vi "北斗显示界面.vi"() -> ()   [LabVIEW 2016, in "环境动力监测库.lvlib" / "NMEA.lvlib"]
uses:
  NMEA.lvlib
  NMEA_GPVTG-data.ctl
  NMEA_Mode.ctl
  NMEA_GPRMC-data.ctl
  NMEA_LatitudeDirection.ctl
  NMEA_LongitudeDirection.ctl
  NMEA_GPGGA-data.ctl
  NMEA_GPS-Quality.ctl
  <vilib>/Utility/miscctls.llb/LVPointTypeDef.ctl
  <vilib>/Instr/_visa.llb/VISA Configure Serial Port (Instr).vi
  <vilib>/Utility/config.llb/NI_LVConfig.lvlib
  <vilib>/ptbypt/NI_PtbyPt.lvlib
panel:
  out "波特率":u32
  out "串口":string
  in  "收方地址设定值":string
  in  "发送测试":bool
  in  "移位报警设定值":dbl=1000.0
  out "浮标定位点":cluster{"纬度":dbl, "经度":dbl}
  out "定位状态":bool
  in  "配置":bool
  out "Coordinates":picture
  in  "reset odometer":bool
  out "方位角 (deg)":dbl(knob) scale=0.0..360.0
  out "偏移量/米":dbl format="%#.2f"
  out "水平运动速度 (km/h)":dbl(knob) scale=0.0..180.0
  out "海拔":dbl format="%.2f"
  out "纬度":dbl
  out "经度":dbl
  out "时间":timestamp format="%<%H:%M:%S>T"
  out "日期":timestamp format="%<%Y/%m/%d>T"
  out "$GPGGA-message_OUT":T1={"TimeStamp"=timestamp(0 s since 1904-01-01), "Latitude"=0.0, "Latitude-Direction"=enum."", "Longitude"=1.0, "Longitude-Direction"=enum."", "GPS-Quality"=enum."GPS fix (SPS)", "Number of Satellites"=0, "Horizontal Dilution of Precision"=0.0, "Altitude above Mean-Sea-Level"=0.0, "Geoidal separation"=0.0, "Time since last DGPS update"=0.0, "DGPS reference station ID"=0} {"Time since last DGPS update" format="%.02f [s]"; "Geoidal separation" format="%.02f [m]"; "Altitude above Mean-Sea-Level" format="%.02f [m]"; "Horizontal Dilution of Precision" format="%.02f [HDOP]"; "Longitude" format="%0.4f [long]"; "Latitude" format="%.04f [lat]"; "TimeStamp" format="%<%.2X>T"}
  out "$GPRMC-message_OUT":T5={"TimeStamp"=timestamp(0 s since 1904-01-01), "Validity"=FALSE, "Latitude"=0.0, "Latitude-Direction"=enum."North", "Longitude"=0.0, "Longitude-Direction"=enum."East", "Speed in knots"=0.0, "True course"=0.0, "Date Stamp"=timestamp(0 s since 1904-01-01), "Magnetic Variation (East/West)"=0.0} {"Magnetic Variation (East/West)" format="%.02f [deg]"; "Date Stamp" format="%<%x>T"; "True course" format="%.02f [deg]"; "Speed in knots" format="%.02f [kts]"; "Longitude" format="%0.4f [long]"; "Latitude" format="%.04f [lat]"; "TimeStamp" format="%<%.2X>T"}
  out "$GPVTG-message_OUT":T6={"True Course over Ground"=0.0, "Magnetic Course over Ground"=0.0, "Speed over Ground in knots"=0.0, "Speed over Ground in km/h"=1.0, "Mode"=""} {"Speed over Ground in km/h" format="%.02f [km/h]"; "Speed over Ground in knots" format="%.02f [kts]"; "Magnetic Course over Ground" format="%.02f [deg]"; "True Course over Ground" format="%.02f [deg]"}
  out "Raw data GPS":string
  in  "Stop":bool
  # "米"
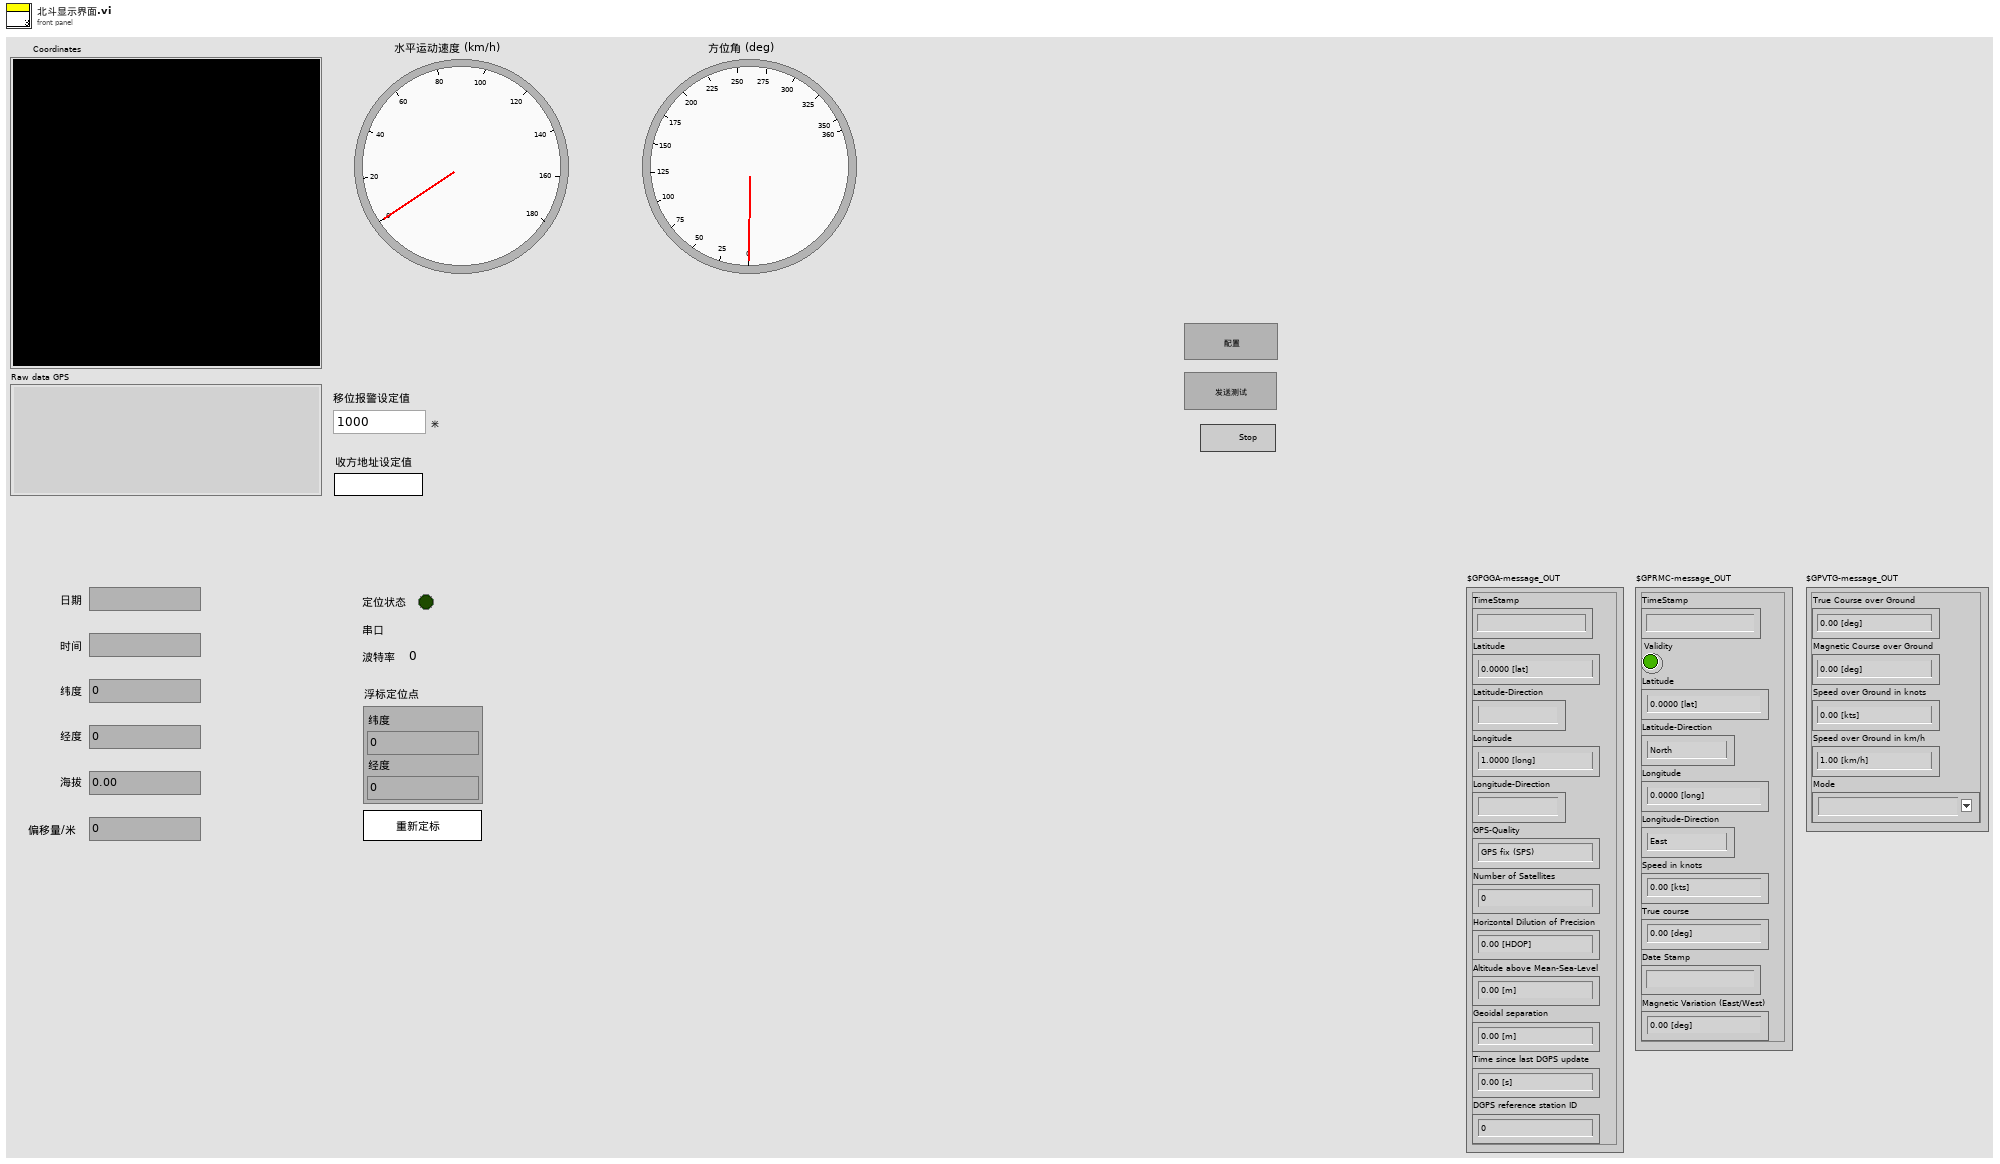
[diagram p1: front panel]
types:
  T1 = typedef "环境动力监测库.lvlib/NMEA.lvlib/NMEA_GPGGA-data.ctl" = cluster{"TimeStamp":timestamp, "Latitude":dbl, "Latitude-Direction":T2, "Longitude":dbl, "Longitude-Direction":T3, "GPS-Quality":T4, "Number of Satellites":i32, "Horizontal Dilution of Precision":dbl, "Altitude above Mean-Sea-Level":dbl, "Geoidal separation":dbl, "Time since last DGPS update":dbl, "DGPS reference station ID":i32}
  T2 = typedef "环境动力监测库.lvlib/NMEA.lvlib/NMEA_LatitudeDirection.ctl" = enum16{"", "North", "South"}
  T3 = typedef "环境动力监测库.lvlib/NMEA.lvlib/NMEA_LongitudeDirection.ctl" = enum16{"", "East", "West"}
  T4 = typedef "环境动力监测库.lvlib/NMEA.lvlib/NMEA_GPS-Quality.ctl" = enum16{"Invalid", "GPS fix (SPS)", "DGPS fix", "PPS fix", "Real Time Kinematic", "Float RTK", "estimated", "Manual input mode", "Simulation mode"}
  T5 = typedef "环境动力监测库.lvlib/NMEA.lvlib/NMEA_GPRMC-data.ctl" = cluster{"TimeStamp":timestamp, "Validity":bool, "Latitude":dbl, "Latitude-Direction":T2, "Longitude":dbl, "Longitude-Direction":T3, "Speed in knots":dbl, "True course":dbl, "Date Stamp":timestamp, "Magnetic Variation (East/West)":dbl}
  T6 = typedef "环境动力监测库.lvlib/NMEA.lvlib/NMEA_GPVTG-data.ctl" = cluster{"True Course over Ground":dbl, "Magnetic Course over Ground":dbl, "Speed over Ground in knots":dbl, "Speed over Ground in km/h":dbl, "Mode":T7}
  T7 = typedef "环境动力监测库.lvlib/NMEA.lvlib/NMEA_Mode.ctl" = string
  T8 = cluster{"监测项描述:输出":string, "连接方式":enum16{"串口", "TCP"}, "端口":string, "IP address:":string, "Port:":string, "站号":u64, "传感器型号":string, "波特率":u64, "data bits":u64, "停止位":u16, "奇偶校验":u16}
  T9 = typedef "LVPointTypeDef.ctl" = cluster{"Horizontal":i16, "Vertical":i16}
  T10 = typedef "NI_LVConfig.lvlib/Config Data RefNum.ctl" = refnum<k1>
  T11 = enum32{"invalid app kind", "Development System", "Run Time System", "Student Edition", "Embedded LabVIEW", "Evaluation", "Custom"}
  T12 = cluster{"电压":dbl, "温度":dbl, "湿度":dbl, "GPS":cluster{"经度":dbl, "纬度":dbl}, "BD":cluster{"经度":dbl, "纬度":dbl}}
  T13 = typedef "LVDateTimeRec.ctl" = cluster{"秒数的小数部分":dbl, "秒":i32, "分":i32, "时":i32, "日":i32, "月":i32, "年":i32, "天数（周）":i32, "天数（年）":i32, "DST":i32}
  T14 = cluster{"温湿度":cluster{"状态":bool, "温度:":sgl, "湿度:":sgl, "详情  ":bool}, "空调":cluster{"状态":bool, "机柜温度:":sgl, "压缩机:":enum16{"停止", "运行"}, "电加热:":enum16{"停止", "运行"}, "详情  ":bool}, "排气扇":cluster{"排气扇:":enum16{"关闭", "打开"}, "详情  ":bool}, "冰箱":cluster{"冰箱:":enum16{"关闭", "打开"}, "详情  ":bool}}
  T15 = cluster{"市电":cluster{"状态":bool, "电压:":u16, "电流：":dbl, "详情  ":bool}, "UPS":cluster{"状态":bool, "输入电压:":sgl, "输出电压:":sgl, "电池电量:":u8, "电量":u16, "详情  ":bool}, "蓄电池12V":cluster{"状态":bool, "电压:":sgl, "电流:":sgl, "电池电量:":u8, "电量":u16, "详情  ":bool}, "蓄电池24V":cluster{"状态":bool, "电压:":sgl, "电流:":sgl, "电池电量:":u8, "电量":u16, "详情  ":bool}}
  T16 = cluster{"网络状态":bool, "电源管理":cluster{"电源管理":bool, "氨氮电源":bool, "总磷电源":bool, "总氮电源":bool, "多参数电源":bool, "CODMn电源":bool, "CODCr电源":bool, "灯带电源":bool, "照明电源":bool}, "北斗-GPS":cluster{"北斗":cluster{"经度:":sgl, "纬度:":sgl, "北斗监测":bool}, "GPS":cluster{"经度:":sgl, "纬度: ":sgl, "GPS监测":bool}}}
  T17 = cluster{"漏水监测输出":cluster{"漏水监测告警":bool, "告警内容":string}, "门禁监测输出":cluster{"门禁监测告警":bool, "告警内容":string}, "门禁监测输出2":cluster{"门禁监测告警":bool, "告警内容":string}, "温湿度监测输出":cluster{"温湿度监测告警":bool, "告警内容":string}, "烟雾监测输出":cluster{"烟雾监测告警":bool, "告警内容":string}, "空调监测输出":cluster{"空调监测告警":bool, "告警内容":string}, "自动重合闸输出":cluster{"自动重合闸告警":bool, "告警内容":string}, "红外入侵输出":cluster{"红外入侵告警":bool, "告警内容":string}, "振动输出":cluster{"振动告警":bool, "告警内容":string}, "UPS输出":cluster{"UPS告警":bool, "告警内容":string}, "蓄电池输出":cluster{"蓄电池告警":bool, "告警内容":string}, "蓄电池输出2":cluster{"蓄电池告警":bool, "告警内容":string}, "GPS输出":cluster{"定位告警":bool, "告警内容":string}, "北斗输出":cluster{"定位告警":bool, "告警内容":string}, "气象输出":cluster{"气象告警":bool, "告警内容":string}}
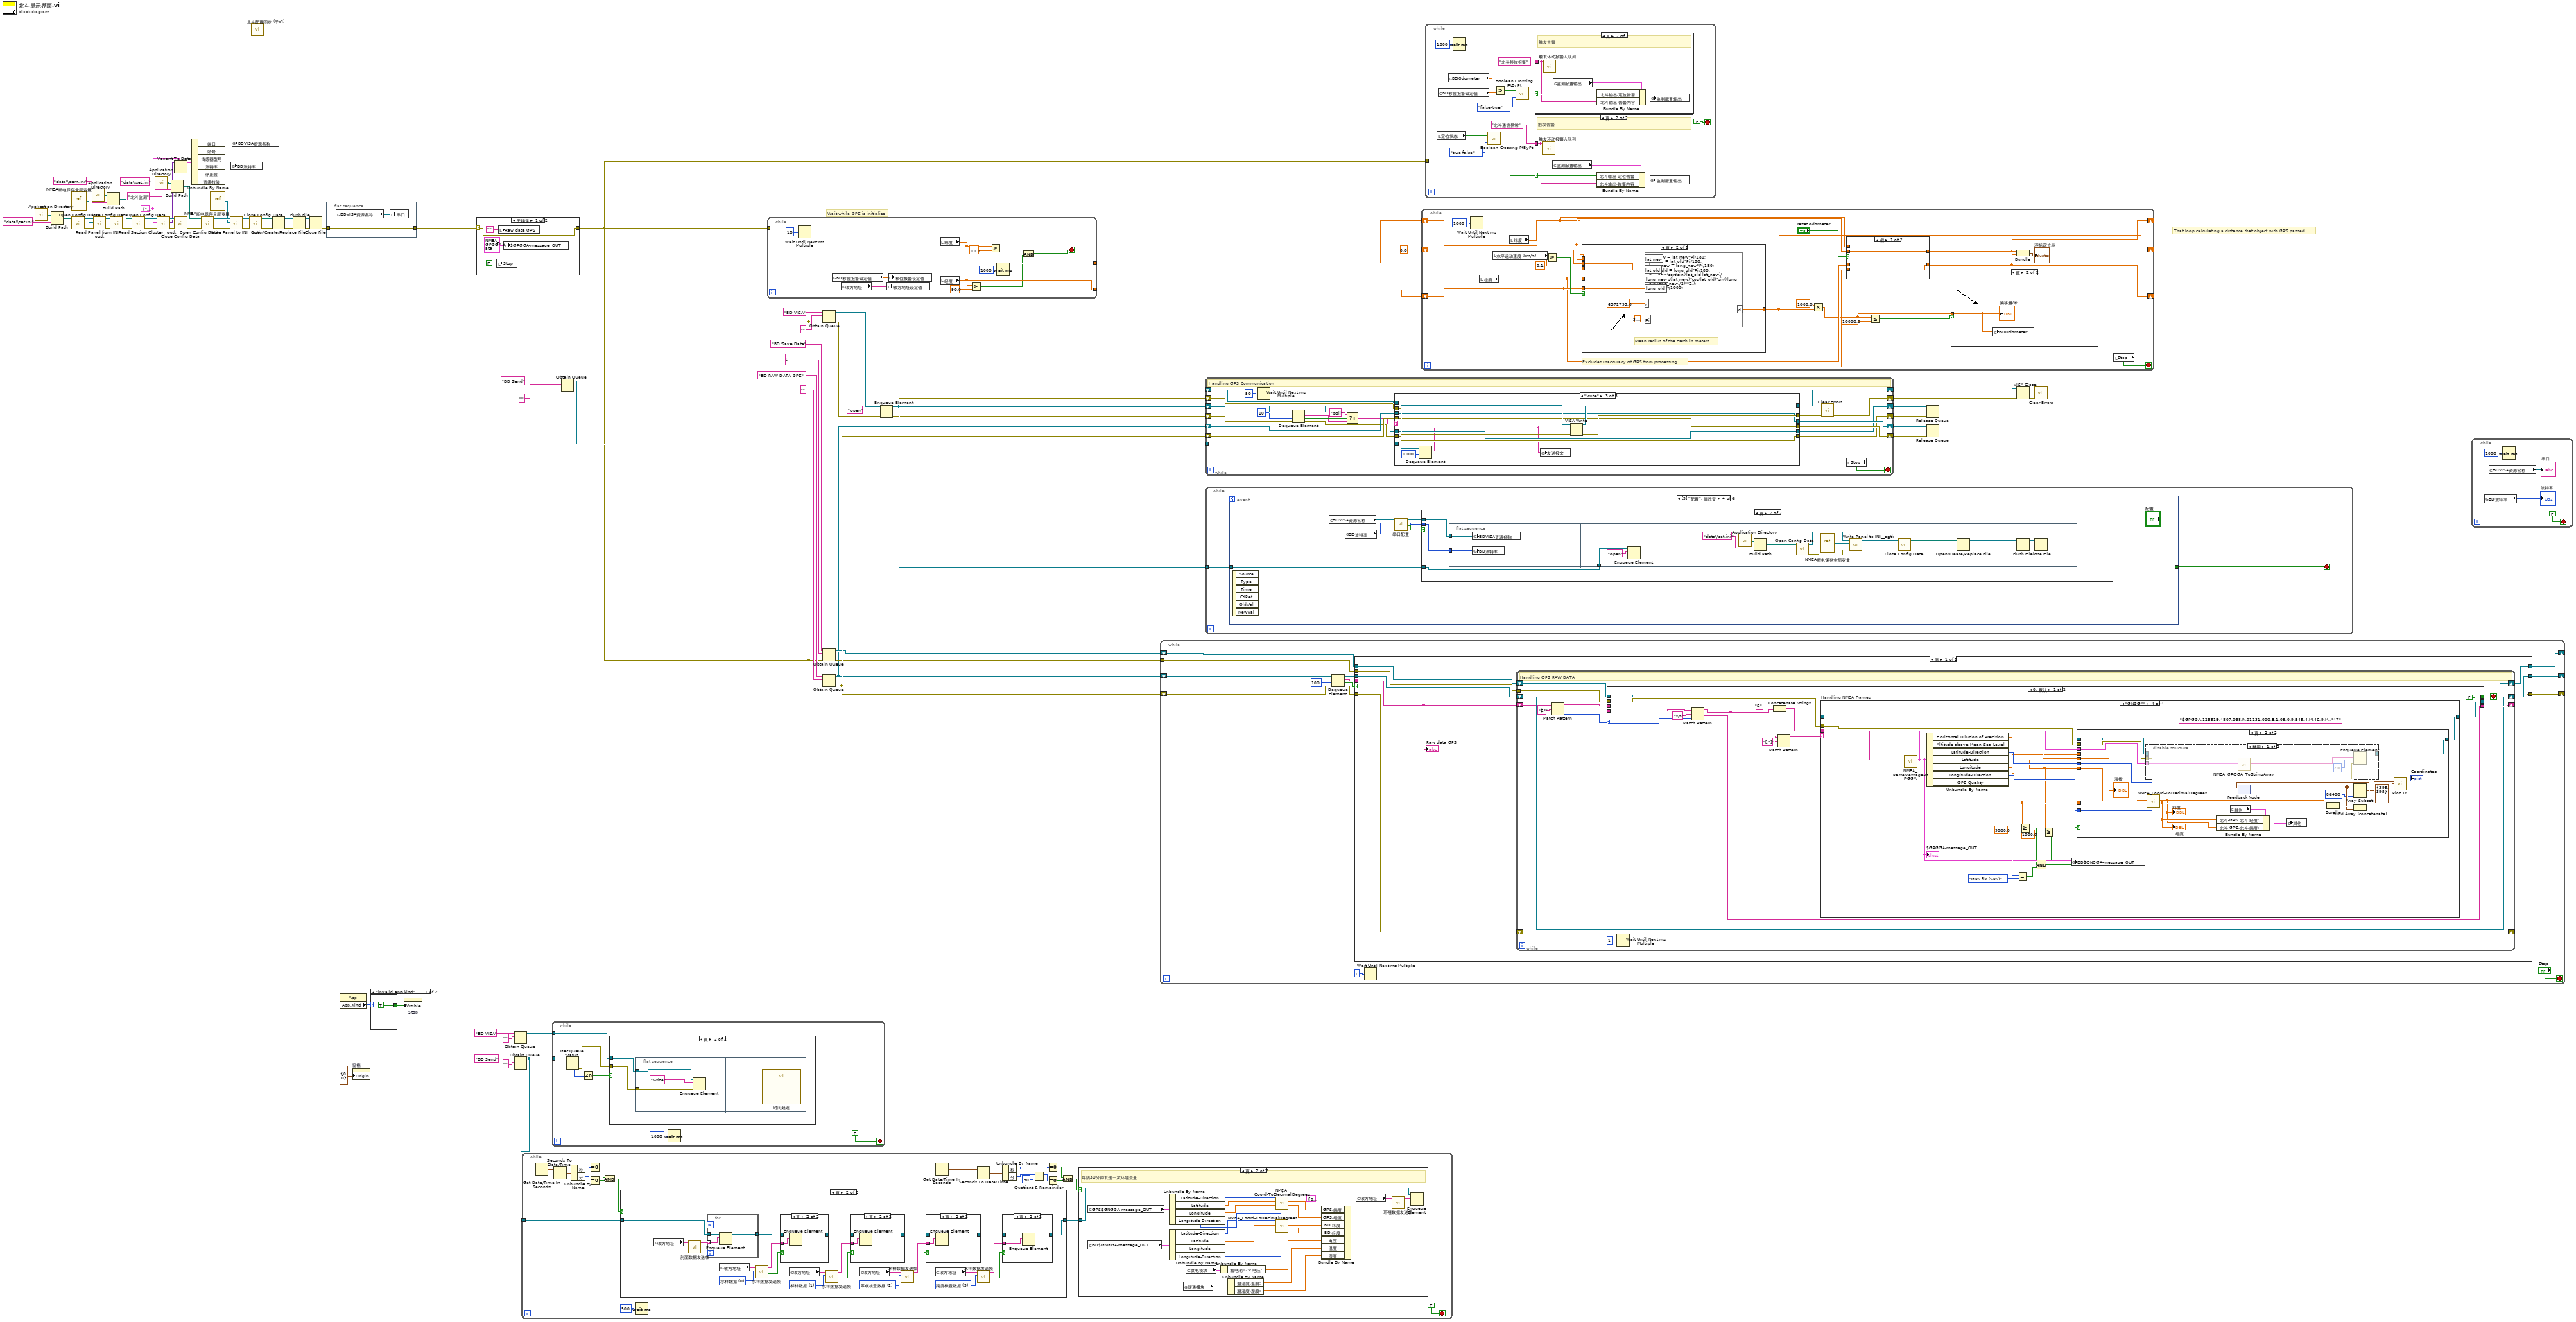
[diagram p0: block diagram]
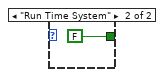
[diagram p11: hidden frame]
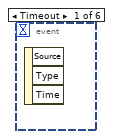
[diagram p12: hidden frame]
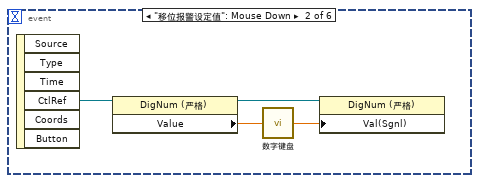
[diagram p13: hidden frame]
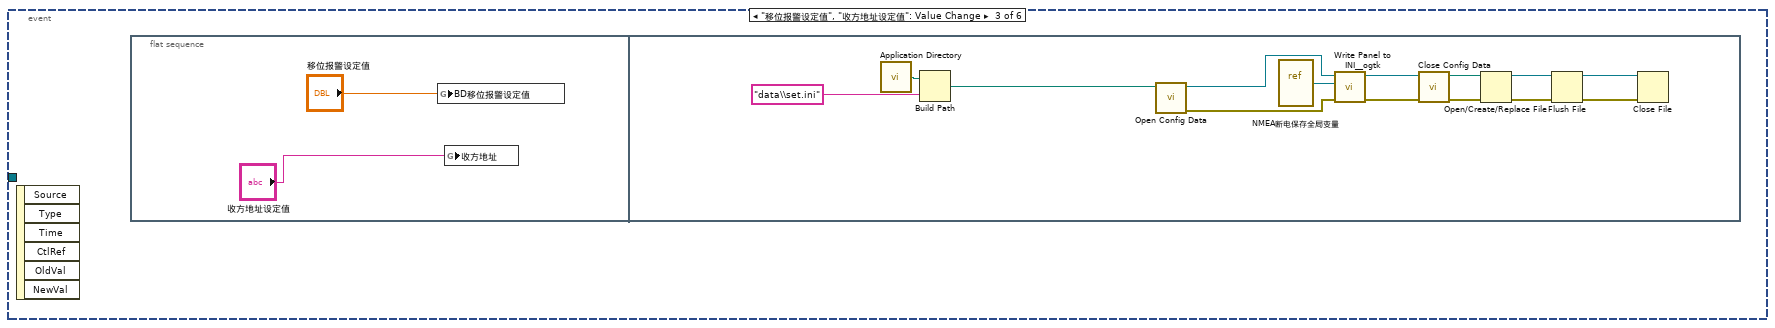
[diagram p14: hidden frame]
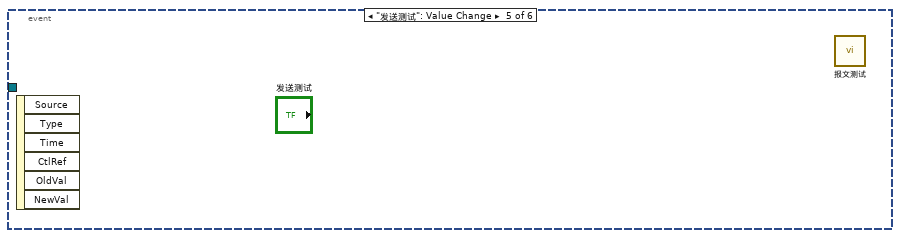
[diagram p16: hidden frame]
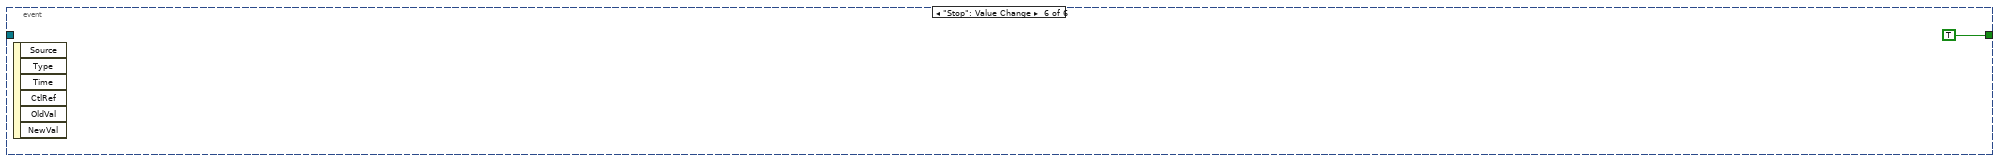
[diagram p17: hidden frame]
diagram:
  w22 = T8 {"监测项描述:输出"="", "连接方式"=enum."串口", "端口"="", "IP address:"="", "Port:"="", "站号"=19200, "传感器型号"="", "波特率"=19200, "data bits"=8, "停止位"=10, "奇偶校验"=0} ("输入簇")
  # "That loop calculating a distance that object with GPS passed"
  # "Wait while GPS is initialize"
  n1 = call <vilib>:"Application Directory.vi"() -> ("Application Directory"=w35:path)
  n2 = Build Path(base path=w35, name or relative path="data\\set.ini" ("名称或相对路径")) -> (appended path=w34:path)
  n3 = vi-ref "NMEA断电保存全局变量.vi"() -> (w33:refnum<vi>)
  n4 = call <vilib>:"Open Config Data.vi"("configuration file path"=w34) -> ("error out"=w38:errorcluster, "refnum"=w37:T10)  [unwired: 8 in, 1 out]
  n5 = call <vilib>:"Application Directory.vi"() -> ("Application Directory"=w29:path)
  n6 = call <userlib>:"Read Panel from INI__ogtk.vi"("error in (no error)"=w38, "VI ref"=w33, "refnum"=w37) -> ("error out"=w40:errorcluster, "refnum out"=w39:T10)  [unwired: 7 in]
  n7 = Build Path(base path=w29, name or relative path="data\\pem.ini" ("名称或相对路径")) -> (appended path=w30:path)
  n8 = call <vilib>:"Close Config Data.vi"("error in (no error)"=w40, "refnum"=w39) -> ("error out"=w4:errorcluster)  [unwired: 8 in, 1 out]
  n9 = call <vilib>:"Open Config Data.vi"("error in (no error)"=w4, "configuration file path"=w30) -> ("error out"=w31:errorcluster, "refnum"=w32:T10)  [unwired: 7 in, 1 out]
  n10 = call <vilib>:"Application Directory.vi"() -> ("Application Directory"=w18:path)
  n11 = call <userlib>:"Read Section Cluster__ogtk.vi"("section (optional)"="北斗监测", "error in (no error)"=w31, "Section Formatted Cluster Type"=w22, "refnum"=w32) -> ("error out"=w25:errorcluster, "Section Formatted Cluster"=w24:variant, "dup refnum"=w26:T10)  [unwired: 3 in, 2 out]
  n12 = Build Path(base path=w18, name or relative path="data\\set.ini" ("名称或相对路径")) -> (appended path=w19:path)
  n13 = Variant To Data(type=w22, Variant=w24) -> (data=w23:T8)  [unwired: 1 in, 1 out]
  n14 = call <vilib>:"Close Config Data.vi"("error in (no error)"=w25, "refnum"=w26) -> ("error out"=w3:errorcluster)  [unwired: 8 in, 1 out]
  n15 = Unbundle By Name(w23) -> ("端口"=w21:string, "波特率"=w20:u64)  [unwired: 4 out]
  n16 = call <vilib>:"Open Config Data.vi"("error in (no error)"=w3, "configuration file path"=w19) -> ("error out"=w15:errorcluster, "refnum"=w16:T10)  [unwired: 7 in, 1 out]
  n17 = vi-ref "NMEA断电保存全局变量.vi"() -> (w12:refnum<vi>)
  n18 = call <userlib>:"Write Panel to INI__ogtk.vi"("error in (no error)"=w15, "VI ref"=w12, "refnum"=w16) -> ("error out"=w13:errorcluster, "refnum out"=w14:T10)  [unwired: 7 in]
  n19 = global write "NMEA断电保存全局变量.vi" "BD波特率"(w20) -> ()
  n20 = global write "NMEA断电保存全局变量.vi" "BDVISA资源名称"(w21) -> ()
  n21 = call <vilib>:"Close Config Data.vi"("error in (no error)"=w13, "refnum"=w14) -> ("error out"=w11:errorcluster, "file path"=w10:path)  [unwired: 8 in]
  n22 = call "北斗配置同步 (子VI).vi"() -> ()  [unwired: 12 in]
  n23 = Open/Create/Replace File(file path (use dialog)=w10, error in=w11) -> (refnum out=w8:refnum<file>, error out=w9:errorcluster)  [unwired: 4 in, 1 out]
  n24 = Flush File(refnum=w8, error in=w9) -> (refnum out=w6:refnum<file>, error out=w7:errorcluster)
  n25 = Close File(refnum=w6, error in=w7) -> (error out=w5:errorcluster)  [unwired: 1 out]
  n26 = flat-sequence {
    tunnel: w5 -> [w78]
    tunnel: [w78] -> w2
    frame #0 {
      n27 = global read "NMEA断电保存全局变量.vi" "BDVISA资源名称"() -> (w79:refnum<visa-resource-name>)
      n28 = local write "串口"(w79) -> ()
    }
  }
  n29 = property class="App"() -> ("App.Kind"=w60:T11)  [unwired: 2 in, 2 out]
  n30 = property on="窗格" class="Pane"("Origin"=T9 {"Horizontal"=0, "Vertical"=0} ("原点")) -> ()  [unwired: 2 in, 2 out]
  n31 = case shown="\"invalid app kind\", 默认" w60 {
    tunnel: [TRUE ("可见") FALSE ("可见")] -> w59
    frame "invalid app kind", Default {
    }
    frame "Run Time System" {
    }
  }
  n32 = property on="Stop" class="Bool (严格)"("Visible"=w59) -> ()  [unwired: 2 in, 2 out]
  n33 = case shown="无错误" w2 {
    selector: w2 -> [w84 w86]
    tunnel: [w84 w86] -> w1
    frame No Error {
      n34 = local write "Stop"(FALSE ("STOP")) -> ()
      n35 = local write "Raw data GPS"("") -> ()
      n36 = local write "$GPGGA-message_OUT"(T1 {"TimeStamp"=timestamp(0 s since 1904-01-01), "Latitude"=0.0, "Latitude-Direction"=enum."North", "Longitude"=0.0, "Longitude-Direction"=enum."East", "GPS-Quality"=enum."Invalid", "Number of Satellites"=0, "Horizontal Dilution of Precision"=0.0, "Altitude above Mean-Sea-Level"=0.0, "Geoidal separation"=0.0, "Time since last DGPS update"=0.0, "DGPS reference station ID"=0} ("GPGGA-data")) -> ()
    }
    frame Error {
    }
  }
  n37 = Obtain Queue(name (unnamed)="BD VISA" ("名称（未命名）"), element data type="" ("名称（未命名）")) -> (queue out=w41:refnum<queue>)  [unwired: 3 in, 2 out]
  n38 = Obtain Queue(name (unnamed)="BD Send" ("名称（未命名）"), element data type="" ("名称（未命名）")) -> (queue out=w44:refnum<queue>)  [unwired: 3 in, 2 out]
  n39 = while {
    tunnel: w44 -> [w106]
    stop <- FALSE stop-if-true
    n40 = Get Date/Time In Seconds() -> (seconds since 1Jan1904=w105:timestamp)
    n41 = Seconds To Date/Time(time stamp (now)=w105) -> (date time rec=w104:T13)  [unwired: 1 in]
    n42 = Unbundle By Name(w104) -> ("秒"=w103:i32, "分"=w102:i32)
    n43 = Equal To 0?(x=w103) -> (x = 0?=w100:bool)
    n44 = Equal To 0?(x=w102) -> (x = 0?=w101:bool)
    n45 = And(x=w100, y=w101) -> (x .and. y?=w98:bool)
    n46 = case shown="真" w98 {
      tunnel: w106 -> [w131 w133]
      tunnel: [w131 w136] -> w89
      frame False {
      }
      frame True {
        w147 = u16 3 items=["水样数据"=0, "标样数据"=1, "零点核查数据"=2, "跨度核查数据"=3, "水样数据补传"=16, "标样核查数据补传"=17, "零点核查数据补传"=18, "跨度核查数据补传"=19] ("数据类别")
        w148 = u16 2 items=["水样数据"=0, "标样数据"=1, "零点核查数据"=2, "跨度核查数据"=3, "水样数据补传"=16, "标样核查数据补传"=17, "零点核查数据补传"=18, "跨度核查数据补传"=19] ("数据类别")
        w151 = u16 1 items=["水样数据"=0, "标样数据"=1, "零点核查数据"=2, "跨度核查数据"=3, "水样数据补传"=16, "标样核查数据补传"=17, "零点核查数据补传"=18, "跨度核查数据补传"=19] ("数据类别")
        w152 = u16 0 items=["水样数据"=0, "标样数据"=1, "零点核查数据"=2, "跨度核查数据"=3, "水样数据补传"=16, "标样核查数据补传"=17, "零点核查数据补传"=18, "跨度核查数据补传"=19] ("数据类别")
        n47 = global read "NMEA断电保存全局变量.vi" "收方地址"() -> (w135:string)
        n48 = call "剖面数据发送帧.vi"("用户地址"=w135) -> ("数据帧"=w134:string[])  [unwired: 10 in]
        n49 = for {
          tunnel: w134 -> [w157] mode=indexing
          tunnel: w133 -> [w158]
          tunnel: [w156] -> w132
          n50 = Enqueue Element(queue=w158, element=w157) -> (queue out=w156:refnum<queue>)  [unwired: 2 in, 2 out]
        }
        n51 = global read "NMEA断电保存全局变量.vi" "收方地址"() -> (w155:string)
        n52 = call "水样数据发送帧.vi"("数据类别"=w152, "用户地址"=w155) -> ("非x？"=w154:bool, "字符串"=w153:string)  [unwired: 7 in, 1 out]
        n53 = case shown="真" w154 {
          tunnel: w153 -> [_ w173]
          tunnel: w132 -> [w171 w174]
          tunnel: [w171 w172] -> w145
          frame False {
          }
          frame True {
            n54 = Enqueue Element(queue=w174, element=w173) -> (queue out=w172:refnum<queue>)  [unwired: 2 in, 2 out]
          }
        }
        n55 = global read "NMEA断电保存全局变量.vi" "收方地址"() -> (w150:string)
        n56 = call "水样数据发送帧.vi"("数据类别"=w151, "用户地址"=w150) -> ("非x？"=w143:bool, "字符串"=w144:string)  [unwired: 7 in, 1 out]
        n57 = case shown="真" w143 {
          tunnel: w144 -> [_ w169]
          tunnel: w145 -> [w167 w170]
          tunnel: [w167 w168] -> w142
          frame False {
          }
          frame True {
            n58 = Enqueue Element(queue=w170, element=w169) -> (queue out=w168:refnum<queue>)  [unwired: 2 in, 2 out]
          }
        }
        n59 = global read "NMEA断电保存全局变量.vi" "收方地址"() -> (w149:string)
        n60 = call "水样数据发送帧.vi"("数据类别"=w148, "用户地址"=w149) -> ("非x？"=w140:bool, "字符串"=w141:string)  [unwired: 7 in, 1 out]
        n61 = case shown="真" w140 {
          tunnel: w141 -> [_ w165]
          tunnel: w142 -> [w163 w166]
          tunnel: [w163 w164] -> w139
          frame False {
          }
          frame True {
            n62 = Enqueue Element(queue=w166, element=w165) -> (queue out=w164:refnum<queue>)  [unwired: 2 in, 2 out]
          }
        }
        n63 = global read "NMEA断电保存全局变量.vi" "收方地址"() -> (w146:string)
        n64 = call "水样数据发送帧.vi"("数据类别"=w147, "用户地址"=w146) -> ("非x？"=w137:bool, "字符串"=w138:string)  [unwired: 7 in, 1 out]
        n65 = case shown="真" w137 {
          tunnel: w138 -> [_ w161]
          tunnel: w139 -> [w159 w162]
          tunnel: [w159 w160] -> w136
          frame False {
          }
          frame True {
            n66 = Enqueue Element(queue=w162, element=w161) -> (queue out=w160:refnum<queue>)  [unwired: 2 in, 2 out]
          }
        }
      }
    }
    n67 = Wait (ms)(milliseconds to wait=u32 500 ("等待时间（毫秒）")) -> ()  [unwired: 1 out]
    n68 = Get Date/Time In Seconds() -> (seconds since 1Jan1904=w94:timestamp)
    n69 = Seconds To Date/Time(time stamp (now)=w94) -> (date time rec=w95:T13)  [unwired: 1 in]
    n70 = Unbundle By Name(w95) -> ("秒"=w96:i32, "分"=w93:i32)
    n71 = Quotient & Remainder(x=w93, y=30) -> (x-y*floor(x/y)=w91:i32)  [unwired: 1 out]
    n72 = Equal To 0?(x=w96) -> (x = 0?=w97:bool)
    n73 = Equal To 0?(x=w91) -> (x = 0?=w90:bool)
    n74 = And(x=w97, y=w90) -> (x .and. y?=w88:bool)
    n75 = case shown="真" w88 {
      tunnel: w89 -> [_ w129]
      frame False {
      }
      frame True {
        # "每隔30分钟发送一次环境变量"
        n76 = global read "NMEA过程全局变量.vi" "GPS$GNGGA-message_OUT"() -> (w124:T1)
        n77 = global read "NMEA过程全局变量.vi" "BD$GNGGA-message_OUT"() -> (w125:T1)
        n78 = Unbundle By Name(w124) -> ("Latitude-Direction"=w121:T2, "Latitude"=w122:dbl, "Longitude"=w123:dbl, "Longitude-Direction"=w120:T3)
        n79 = Unbundle By Name(w125) -> ("Latitude-Direction"=w115:T2, "Latitude"=w117:dbl, "Longitude"=w116:dbl, "Longitude-Direction"=w114:T3)
        n80 = global read "内部交互全局变量.vi" "暖通模块"() -> (w110:T14)
        n81 = global read "内部交互全局变量.vi" "供电模块"() -> (w111:T15)
        n82 = Unbundle By Name(w111) -> ("蓄电池12V.电压:"=w109:sgl)
        n83 = Unbundle By Name(w110) -> ("温湿度.温度:"=w108:sgl, "温湿度.湿度:"=w107:sgl)
        n84 = call "NMEA_Coord-ToDecimalDegrees.vi"("Longitude-Direction"=w120, "Latitude-Direction"=w121, "Longitude"=w123, "Latitude"=w122) -> ("Longitude"=w118:dbl, "Latitude"=w119:dbl)  [unwired: 6 in]
        n85 = call "NMEA_Coord-ToDecimalDegrees.vi"("Longitude-Direction"=w114, "Latitude-Direction"=w115, "Longitude"=w116, "Latitude"=w117) -> ("Longitude"=w112:dbl, "Latitude"=w113:dbl)  [unwired: 6 in]
        n86 = Bundle By Name(cluster=T12 {"电压"=0.0, "温度"=0.0, "湿度"=0.0, "GPS"={"经度"=0.0, "纬度"=0.0}, "BD"={"经度"=0.0, "纬度"=0.0}} ("环境变量"), "GPS.纬度"=w119, "GPS.经度"=w118, "BD.纬度"=w113, "BD.经度"=w112, "电压"=w109, "温度"=w108, "湿度"=w107) -> (w126:T12)
        n87 = global read "NMEA断电保存全局变量.vi" "收方地址"() -> (w130:string)
        n88 = call "环境数据发送帧.vi"("环境变量"=w126, "用户地址"=w130) -> ("字符串"=w128:string)  [unwired: 8 in, 1 out]
        n89 = Enqueue Element(queue=w129, element=w128) -> ()  [unwired: 2 in, 3 out]
      }
    }
  }
  n90 = while {
    tunnel: w44 -> [w180]
    tunnel: w41 -> [w181]
    stop <- FALSE stop-if-true
    n91 = Get Queue Status(queue=w180) -> (error out=w179:errorcluster, # elements in queue=w177:i32)  [unwired: 2 in, 6 out]
    n92 = Not Equal To 0?(x=w177) -> (x != 0?=w176:bool)
    n93 = case shown="真" w176 {
      tunnel: w181 -> [_ w183]
      tunnel: w179 -> [_ w182]
      frame False {
      }
      frame True {
        n94 = flat-sequence {
          tunnel: w183 -> [w186]
          tunnel: w182 -> [w185]
          frame #0 {
            n95 = Enqueue Element(queue=w186, element="write" ("元素"), error in (no error)=w185) -> ()  [unwired: 1 in, 3 out]
          }
          frame #1 {
            n96 = call "时间延迟"() -> ()  [unwired: 11 in, 1 out]
          }
        }
      }
    }
    n97 = Wait (ms)(milliseconds to wait=u32 1000 ("等待时间（毫秒）")) -> ()  [unwired: 1 out]
  }
  n98 = Obtain Queue(name (unnamed)="BD Send" ("名称（未命名）"), element data type="" ("名称（未命名）")) -> (queue out=w47:refnum<queue>)  [unwired: 3 in, 2 out]
  n99 = while {
    tunnel: [w191] -> w62
    tunnel: [w193] -> w63
    tunnel: w1 -> [_]
    stop <- w187 stop-if-true
    n100 = Wait Until Next ms Multiple(millisecond multiple=u32 10) -> ()  [unwired: 1 out]
    n101 = global read "NMEA断电保存全局变量.vi" "BD移位报警设定值"() -> (w196:dbl)
    n102 = global read "NMEA断电保存全局变量.vi" "收方地址"() -> (w195:string)
    n103 = local write "收方地址设定值"(w195) -> ()
    n104 = local write "移位报警设定值"(w196) -> ()
    n105 = local read "纬度"() -> (w193:dbl)
    n106 = local read "经度"() -> (w191:dbl)
    n107 = Greater Or Equal?(x=w191, y=90.0) -> (x >= y?=w188:bool)
    n108 = Greater Or Equal?(x=w193, y=10.0) -> (x >= y?=w189:bool)
    n109 = Wait (ms)(milliseconds to wait=u32 1000 ("等待时间（毫秒）")) -> ()  [unwired: 1 out]
    n110 = And(x=w189, y=w188) -> (x .and. y?=w187:bool)
  }
  n111 = Obtain Queue(name (unnamed)="BD VISA" ("名称（未命名）"), element data type="" ("名称（未命名）"), error in (no error)=w1) -> (queue out=w56:refnum<queue>, error out=w54:errorcluster)  [unwired: 2 in, 1 out]
  n112 = Obtain Queue(name (unnamed)="BD Save Data" ("名称（未命名）"), element data type=string[] [], error in (no error)=w1) -> (queue out=w76:refnum<queue>, error out=w75:errorcluster)  [unwired: 2 in, 1 out]
  n113 = Obtain Queue(name (unnamed)="BD RAW DATA GPS" ("nom (aucun)"), element data type="" ("expression régulière"), error in (no error)=w1) -> (queue out=w70:refnum<queue>, error out=w77:errorcluster)  [unwired: 2 in, 1 out]
  n114 = Enqueue Element(queue=w56, element="open" ("元素"), error in (no error)=w54) -> (queue out=w55:refnum<queue>, error out=w53:errorcluster)  [unwired: 1 in, 1 out]
  n115 = while {
    tunnel: w75 -> [w207]
    shift-right: [w205] -> _
    shift-left: w70 -> [w206]
    shift-right: [w201] -> _
    shift-left: w76 -> [w208]
    shift-right: [w200] -> _
    shift-left: w77 -> [w211]
    stop <- "Stop" stop-if-true
    n116 = Dequeue Element(queue=w206, timeout in ms (-1)=100 ("timeout en ms (-1)"), error in (no error)=w211) -> (queue out=w204:refnum<queue>, element=w210:string, timed out?=w202:bool, error out=w199:errorcluster)
    n117 = case shown="假" w202 {
      tunnel: w210 -> [w212 _]
      tunnel: w208 -> [w219 w326]
      tunnel: w207 -> [w218 _]
      tunnel: [w217 w327] -> w205
      tunnel: w204 -> [w216 w327]
      tunnel: [w215 w326] -> w201
      tunnel: [w214 w325] -> w200
      tunnel: w199 -> [w213 w325]
      frame False {
        n118 = while {
          shift-right: [w230] -> _
          shift-left: w212 -> [w221]
          tunnel: w218 -> [w227]
          shift-right: [w226] -> w217
          shift-left: w216 -> [w226]
          shift-right: [w224] -> w215
          shift-left: w219 -> [w228]
          shift-right: [w223] -> w214
          shift-left: w213 -> [w223]
          stop <- w225 stop-if-true
          # "Handling GPS RAW DATA"
          n119 = Match Pattern(string=w221, regular expression="$*" ("expression régulière")) -> (before substring=w222:string, after substring=w220:string, offset past match=w231:i32)  [unwired: 1 in, 1 out]
          n120 = case shown="0, 默认" w231 {
            selector: w231 -> [w245 _]
            tunnel: [w244 w322] -> w230
            tunnel: w220 -> [w236 _]
            tunnel: [FALSE TRUE] -> w225
            tunnel: w228 -> [w242 w323]
            tunnel: w227 -> [w241 _]
            tunnel: [w239 w323] -> w224
            tunnel: w222 -> [_ w322]
            frame 0, Default {
              n121 = Match Pattern(string=w236, regular expression="\\n" ("expression régulière"), offset (0)=w245) -> (before substring=w235:string, after substring=w244:string)  [unwired: 2 out]
              n122 = Concatenate Strings("$" ("expression régulière"), w235) -> (w234:string)
              n123 = Match Pattern(string=w235, regular expression="[,*]" ("正则表达式")) -> (before substring=w237:string)  [unwired: 1 in, 3 out]
              n124 = case "Handling NMEA Frames" shown="\"GNGGA\"" w237 {
                selector: w237 -> [w248 _ _ _]
                tunnel: w234 -> [w249 w265 w273 w294]
                tunnel: w242 -> [w250 w264 w272 w291]
                tunnel: w241 -> [_ _ _ w290]
                tunnel: [w250 w264 w272 w289] -> w239
                frame " ", Default {
                  n125 = String Subset(string=w248, length (rest)=4 ("长度（剩余）")) -> (substring=w246:string)  [unwired: 1 in]
                  n126 = case shown="\"FKXX\", \"ICJC\", \"ICXX\", \"TXSQ\", \"TXXX\"" w246 {
                    tunnel: w249 -> [_ w257]
                    frame "假", Default {
                    }
                    frame "FKXX", "ICJC", "ICXX", "TXSQ", "TXXX" {
                      n127 = Search/Split String(string=w257, search string/char (-)="GP" ("搜索字符串/字符(-)")) -> (substring before match=w255:string)  [unwired: 1 in, 2 out]
                      n128 = Search/Split String(string=w255, search string/char (-)="GN" ("搜索字符串/字符(-)")) -> (substring before match=w252:string)  [unwired: 1 in, 2 out]
                      n129 = Search/Split String(string=w252, search string/char (-)="BD" ("搜索字符串/字符(-)")) -> (substring before match=w251:string)  [unwired: 1 in, 2 out]
                      n130 = global write "发送报文全局变量.vi" "接收命令"(w251) -> ()
                    }
                  }
                }
                frame "GNVTG" {
                  (unwired) "$GPVTG,054.7,T,034.4,M,005.5,N,010.2,K*48" ("$GPVTG-message_IN")
                  n131 = call "NMEA_ParseMessage-GPVTG.vi"("$GPVTG-message_IN"=w265) -> ("$GPVTG-message_OUT"=w263:T6)  [unwired: 9 in, 1 out]
                  "$GPVTG-message_OUT" <- w263
                  n132 = Unbundle By Name(w263) -> ("True Course over Ground"=w259:dbl, "Speed over Ground in km/h"=w258:dbl, "Mode"=w262:T7)
                  n133 = Not Equal?(x=w262, y=T7 "N" ("Mode")) -> (x != y?=w260:bool)
                  n134 = case shown="真" w260 {
                    tunnel: w259 -> [_ w266]
                    tunnel: w258 -> [_ w267]
                    frame False {
                    }
                    frame True {
                      "水平运动速度 (km/h)" <- w267
                      "方位角 (deg)" <- w266
                    }
                  }
                }
                frame "GNRMC" {
                  (unwired) "$GPRMC,225446,A,4916.45,N,12311.12,W,000.5,054.7,191194,020.3,E*68" ("$GPRMC-message_IN")
                  n135 = call "NMEA_ParseMessage-GPRMC.vi"("$GPRMC-message_IN"=w273) -> ("$GPRMC-message_OUT"=w271:T5)  [unwired: 9 in, 1 out]
                  "$GPRMC-message_OUT" <- w271
                  n136 = Unbundle By Name(w271) -> ("Validity"=w270:bool, "TimeStamp"=w269:timestamp, "Date Stamp"=w268:timestamp)
                  "定位状态" <- w270
                  n137 = case shown="真" w270 {
                    tunnel: w269 -> [_ w274]
                    tunnel: w268 -> [_ w275]
                    frame False {
                    }
                    frame True {
                      "时间" <- w274
                      "日期" <- w275
                    }
                  }
                }
                frame "GNGGA" {
                  (unwired) "$GPGGA,123519,4807.038,N,01131.000,E,1,08,0.9,545.4,M,46.9,M,,*47" ("data out")
                  n138 = call "NMEA_ParseMessage-GPGGA.vi"("$GPGGA-message_IN"=w294) -> ("$GPGGA-message_OUT"=w282:T1)  [unwired: 9 in, 1 out]
                  "$GPGGA-message_OUT" <- w282
                  n139 = Unbundle By Name(w282) -> ("Horizontal Dilution of Precision"=w283:dbl, "Altitude above Mean-Sea-Level"=w284:dbl, "Latitude-Direction"=w292:T2, "Latitude"=w279:dbl, "Longitude"=w281:dbl, "Longitude-Direction"=w293:T3, "GPS-Quality"=w285:T4)
                  n140 = Equal?(x=w285, y=NMEA_GPS-Quality."GPS fix (SPS)" ("GPS-Quality")) -> (x = y?=w286:bool)
                  n141 = Greater Or Equal?(x=w281, y=9000.0) -> (x >= y?=w277:bool)
                  n142 = Greater Or Equal?(x=w279, y=1000.0) -> (x >= y?=w276:bool)
                  n143 = Compound Arithmetic op=AND(w276, w277, w286) -> (w288:bool)
                  n144 = global write "NMEA过程全局变量.vi" "BD$GNGGA-message_OUT"(w282) -> ()
                  n145 = case shown="真" w288 {
                    tunnel: w293 -> [_ w315]
                    tunnel: w279 -> [_ w309]
                    tunnel: w292 -> [_ w308]
                    tunnel: w282 -> [_ w314]
                    tunnel: w291 -> [w295 w313]
                    tunnel: w290 -> [_ w312]
                    tunnel: [w295 w311] -> w289
                    tunnel: w281 -> [_ w310]
                    tunnel: w284 -> [_ w307]
                    tunnel: w283 -> [_ _]
                    frame False {
                    }
                    frame True {
                      n146 = disable-structure shown="禁用" {
                        disable-tunnel: w314 -> [w321 _]
                        disable-tunnel: w313 -> [w320 _]
                        disable-tunnel: w312 -> [w319 _]
                        disable-tunnel: [w317 _] -> w311
                        frame Disabled {
                          n147 = call "NMEA_GPGGA_ToStringArray.vi"("$GPGGA-message_IN"=w321) -> ("$GPGGA-message_OUT"=w318:string[])  [unwired: 9 in, 1 out]
                          n148 = Enqueue Element(queue=w320, element=w318, timeout in ms (-1)=20 ("timeout en ms (-1)"), error in (no error)=w319) -> (queue out=w317:refnum<queue>)  [unwired: 2 out]
                        }
                        frame Enabled {
                        }
                      }
                      n149 = call "NMEA_Coord-ToDecimalDegrees.vi"("Longitude-Direction"=w315, "Latitude-Direction"=w308, "Longitude"=w310, "Latitude"=w309) -> ("Longitude"=w297:dbl, "Latitude"=w296:dbl)  [unwired: 6 in]
                      "经度" <- w297
                      "纬度" <- w296
                      n150 = global read "内部交互全局变量.vi" "其他"() -> (w298:T16)
                      n151 = Bundle By Name(cluster=w298, "北斗-GPS.北斗.经度:"=w297, "北斗-GPS.北斗.纬度:"=w296) -> (w299:T16)
                      n152 = feedback #1() -> (w302:cluster{"Longitude":dbl, "Latitude":dbl}[])  [unwired: 1 in]
                      n153 = global write "内部交互全局变量.vi" "其他"(w299) -> ()
                      n154 = Bundle("Longitude"=w297, "Latitude"=w296) -> (w304:cluster{"Longitude":dbl, "Latitude":dbl})  [unwired: 1 in]
                      n155 = Array Subset(array=w302, length=86400 ("长度")) -> (w303:cluster{"Longitude":dbl, "Latitude":dbl}[])  [unwired: 1 in]
                      n156 = Build Array (concatenate)(w304, w302) -> (w306:cluster{"Longitude":dbl, "Latitude":dbl}[])
                      n157 = feedback-in #1(w306) -> ()
                      n158 = call <vilib>:"Plot XY.vi"("data"=w303, "dimensions (w,h)"=cluster{"width":i16, "height":i16} {"width"=395, "height"=395}) -> ("new picture"=→"Coordinates":picture)  [unwired: 13 in]
                      "海拔" <- w307
                    }
                  }
                }
              }
            }
            frame -1 {
            }
          }
          n159 = Wait Until Next ms Multiple(millisecond multiple=u32 1 ("n millisecondes")) -> ()  [unwired: 1 out]
        }
        "Raw data GPS" <- w212
      }
      frame True {
      }
    }
    n160 = Wait Until Next ms Multiple(millisecond multiple=u32 1 ("n millisecondes")) -> ()  [unwired: 1 out]
  }
  n161 = while {
    shift-right: [w347] -> w72
    shift-left: w77 -> [w349]
    shift-right: [w346] -> w69
    shift-left: _ -> [w345]
    shift-right: [w348] -> w71
    shift-left: w70 -> [w350]
    shift-right: [w341] -> w68
    shift-left: w1 -> [w343]
    shift-right: [w330] -> w51
    shift-left: w53 -> [w338]
    shift-right: [w332] -> w50
    shift-left: w55 -> [w339]
    tunnel: w47 -> [w328]
    stop <- w340 stop-if-true
    # "Handling GPS Communication"
    n162 = Wait Until Next ms Multiple(millisecond multiple=u32 50 ("attente (ms)")) -> ()  [unwired: 1 out]
    n163 = Dequeue Element(queue=w339, timeout in ms (-1)=10 ("超时毫秒(-1)"), error in (no error)=w338) -> (queue out=w331:refnum<queue>, element=w334:string, timed out?=w336:bool, error out=w329:errorcluster)
    n164 = Select(t="poll" ("名称（未命名）"), s=w336, f=w334) -> (s? t:f=w333:string)
    n165 = case shown="\"write\"" w333 {
      tunnel: w350 -> [w362 w377 w396]
      tunnel: w349 -> [w361 w376 w399]
      tunnel: [w362 w375 w396] -> w348
      tunnel: [w361 w374 w399] -> w347
      tunnel: [w353 w373 w402] -> w346
      tunnel: w345 -> [w356 w372 w403]
      tunnel: w343 -> [w357 w371 w400]
      tunnel: [w351 w370 w401] -> w342
      tunnel: [w364 w366 w397] -> w332
      tunnel: w331 -> [w364 w366 w397]
      tunnel: [w363 w365 w398] -> w330
      tunnel: w329 -> [w363 w365 w398]
      tunnel: w328 -> [_ _ w395]
      frame "open" {
        n166 = VISA Close(VISA resource name=w356, error in (no error)=w357) -> (error out=w355:errorcluster)
        n167 = call <vilib>:"Clear Errors.vi"("error in (no error)"=w355) -> ("error out"=w354:errorcluster)  [unwired: 5 in, 1 out]
        n168 = global read "NMEA断电保存全局变量.vi" "BDVISA资源名称"() -> (w359:refnum<visa-resource-name>)
        n169 = global read "NMEA断电保存全局变量.vi" "BD波特率"() -> (w360:u32)
        n170 = call-poly "VISA Configure Serial Port"("VISA resource name"=w359, "baud rate (9600)"=w360, "error in (no error)"=w354) -> ("VISA resource name out"=w358:refnum<visa-resource-name>, "error out"=w352:errorcluster)  [unwired: 11 in]
        n171 = VISA Clear(VISA resource name=w358, error in (no error)=w352) -> (VISA resource name out=w353:refnum<visa-resource-name>, error out=w351:errorcluster)
      }
      frame "poll", Default {
        n172 = property class="Instr"(reference=w372, error in=w371) -> (reference out=w369:refnum<visa-resource-name>, error out=w368:errorcluster, "Bytes at Port"=w367:u32)
        n173 = case shown="1, 默认" w367 {
          selector: w367 -> [_ w383]
          tunnel: w377 -> [w378 w392]
          tunnel: w376 -> [w379 w391]
          tunnel: [w378 w390] -> w375
          tunnel: [w379 w389] -> w374
          tunnel: [w380 w387] -> w373
          tunnel: w369 -> [w380 w386]
          tunnel: w368 -> [w381 w385]
          tunnel: [w381 w384] -> w370
          frame 0 {
          }
          frame 1, Default {
            n174 = VISA Read(VISA resource name=w386, byte count=w383, error in (no error)=w385) -> (VISA resource name out=w387:refnum<visa-resource-name>, read buffer=w388:string, error out=w384:errorcluster)  [unwired: 1 out]
            n175 = Enqueue Element(queue=w392, element=w388, timeout in ms (-1)=20 ("timeout en ms (-1)"), error in (no error)=w391) -> (queue out=w390:refnum<queue>, error out=w389:errorcluster)  [unwired: 1 out]
          }
        }
      }
      frame "write" {
        n176 = Dequeue Element(queue=w395, timeout in ms (-1)=1000 ("超时毫秒(-1)")) -> (element=w393:string)  [unwired: 1 in, 3 out]
        n177 = global write "发送报文全局变量.vi" "发送报文"(w393) -> ()
        n178 = VISA Write(VISA resource name=w403, write buffer=w393, error in (no error)=w400) -> (VISA resource name out=w402:refnum<visa-resource-name>, error out=w401:errorcluster)  [unwired: 1 out]
      }
    }
    n179 = call <vilib>:"Clear Errors.vi"("error in (no error)"=w342) -> ("error out"=w341:errorcluster)  [unwired: 5 in, 1 out]
    n180 = local read "Stop"() -> (w340:bool)
  }
  n181 = while {
    tunnel: w55 -> [w404]
    stop <- w405 stop-if-true
    n182 = event shown="[3] \"配置\": 值改变" {
      selector: _ -> [_ _ _ _ _ _]
      dyn-events: _ -> [_ _ _ _ _ _]
      timeout: _ -> [_ _ _ _ _ _]
      tunnel: [_ _ _ _ _ TRUE] -> w405
      tunnel: w404 -> [_ _ _ w426 _ _]
      event Timeout {
        n183 = event-data() -> ()  [unwired: 1 in, 3 out]
      }
      event "移位报警设定值": Mouse Down {
        n184 = event-data() -> ("CtlRef"=w409:refnum<vi>)  [unwired: 1 in, 5 out]
        n185 = property class="DigNum (严格)"(reference=w409) -> (reference out=w406:refnum<vi>, "Value"=w408:dbl)  [unwired: 1 in, 1 out]
        n186 = call "数字键盘.vi"("OldNumber"=w408) -> ("NewNumber"=w407:dbl)
        n187 = property class="DigNum (严格)"(reference=w406, "Val(Sgnl)"=w407) -> ()  [unwired: 1 in, 2 out]
      }
      event "移位报警设定值", "收方地址设定值": Value Change {
        n188 = event-data() -> ()  [unwired: 1 in, 6 out]
        n189 = flat-sequence {
          frame #0 {
            n190 = global write "NMEA断电保存全局变量.vi" "BD移位报警设定值"("移位报警设定值") -> ()
            n191 = global write "NMEA断电保存全局变量.vi" "收方地址"("收方地址设定值") -> ()
          }
          frame #1 {
            n192 = call <vilib>:"Application Directory.vi"() -> ("Application Directory"=w424:path)
            n193 = Build Path(base path=w424, name or relative path="data\\set.ini" ("名称或相对路径")) -> (appended path=w425:path)
            n194 = call <vilib>:"Open Config Data.vi"("configuration file path"=w425) -> ("error out"=w421:errorcluster, "refnum"=w422:T10)  [unwired: 8 in, 1 out]
            n195 = vi-ref "NMEA断电保存全局变量.vi"() -> (w418:refnum<vi>)
            n196 = call <userlib>:"Write Panel to INI__ogtk.vi"("error in (no error)"=w421, "VI ref"=w418, "refnum"=w422) -> ("error out"=w419:errorcluster, "refnum out"=w420:T10)  [unwired: 7 in]
            n197 = call <vilib>:"Close Config Data.vi"("error in (no error)"=w419, "refnum"=w420) -> ("error out"=w417:errorcluster, "file path"=w416:path)  [unwired: 8 in]
            n198 = Open/Create/Replace File(file path (use dialog)=w416, error in=w417) -> (refnum out=w414:refnum<file>, error out=w415:errorcluster)  [unwired: 4 in, 1 out]
            n199 = Flush File(refnum=w414, error in=w415) -> (refnum out=w412:refnum<file>, error out=w413:errorcluster)
            n200 = Close File(refnum=w412, error in=w413) -> ()  [unwired: 2 out]
          }
        }
      }
      event "配置": Value Change {
        n201 = event-data() -> ()  [unwired: 1 in, 6 out]
        n202 = global read "NMEA断电保存全局变量.vi" "BDVISA资源名称"() -> (w429:refnum<visa-resource-name>)
        n203 = global read "NMEA断电保存全局变量.vi" "BD波特率"() -> (w427:u32)
        n204 = call "串口配置.vi"("波特率"=w427, "VISA资源名称"=w429) -> ("确认 2"=w431:bool, "波特率输出"=w428:u32, "VISA资源名称 2"=w430:refnum<visa-resource-name>)  [unwired: 7 in]
        n205 = case shown="真" w431 {
          tunnel: w430 -> [_ w434]
          tunnel: w428 -> [_ w433]
          tunnel: w426 -> [_ w432]
          frame False {
          }
          frame True {
            n206 = flat-sequence {
              tunnel: w434 -> [w436]
              tunnel: w433 -> [w435]
              tunnel: w432 -> [w438]
              frame #0 {
                n207 = global write "NMEA断电保存全局变量.vi" "BDVISA资源名称"(w436) -> ()
                n208 = global write "NMEA断电保存全局变量.vi" "BD波特率"(w435) -> ()
              }
              frame #1 {
                n209 = Enqueue Element(queue=w438, element="open" ("元素")) -> ()  [unwired: 2 in, 3 out]
                n210 = call <vilib>:"Application Directory.vi"() -> ("Application Directory"=w451:path)
                n211 = Build Path(base path=w451, name or relative path="data\\set.ini" ("名称或相对路径")) -> (appended path=w452:path)
                n212 = call <vilib>:"Open Config Data.vi"("configuration file path"=w452) -> ("error out"=w448:errorcluster, "refnum"=w449:T10)  [unwired: 8 in, 1 out]
                n213 = vi-ref "NMEA断电保存全局变量.vi"() -> (w445:refnum<vi>)
                n214 = call <userlib>:"Write Panel to INI__ogtk.vi"("error in (no error)"=w448, "VI ref"=w445, "refnum"=w449) -> ("error out"=w446:errorcluster, "refnum out"=w447:T10)  [unwired: 7 in]
                n215 = call <vilib>:"Close Config Data.vi"("error in (no error)"=w446, "refnum"=w447) -> ("error out"=w444:errorcluster, "file path"=w443:path)  [unwired: 8 in]
                n216 = Open/Create/Replace File(file path (use dialog)=w443, error in=w444) -> (refnum out=w441:refnum<file>, error out=w442:errorcluster)  [unwired: 4 in, 1 out]
                n217 = Flush File(refnum=w441, error in=w442) -> (refnum out=w439:refnum<file>, error out=w440:errorcluster)
                n218 = Close File(refnum=w439, error in=w440) -> ()  [unwired: 2 out]
              }
            }
          }
        }
      }
      event "发送测试": Value Change {
        n219 = event-data() -> ()  [unwired: 1 in, 6 out]
        n220 = call "报文测试.vi"() -> ()  [unwired: 12 in]
      }
      event "Stop": Value Change {
        n221 = event-data() -> ()  [unwired: 1 in, 6 out]
      }
    }
  }
  n222 = while {
    shift-right: [w470] -> _
    shift-left: 0.0 -> [w466]
    shift-right: [w461] -> _
    shift-left: w62 -> [w464]
    shift-right: [w462] -> _
    shift-left: w63 -> [w463]
    stop <- w469 stop-if-true
    # "Excludes inaccuracy of GPS from processing"
    n223 = Wait Until Next ms Multiple(millisecond multiple=u32 1000 ("Refresh period (ms)")) -> ()  [unwired: 1 out]
    n224 = local read "经度"() -> (w458:dbl)
    n225 = local read "水平运动速度 (km/h)"() -> (w459:dbl)
    n226 = local read "纬度"() -> (w457:dbl)
    n227 = Greater Or Equal?(x=w459, y=0.1) -> (x >= y?=w472:bool)
    n228 = case shown="真" w472 {
      tunnel: w464 -> [_ w483]
      tunnel: w463 -> [_ w481]
      tunnel: w457 -> [_ w480]
      tunnel: w458 -> [_ w482]
      tunnel: w466 -> [w478 _]
      tunnel: [w478 w479] -> w470
      frame False {
      }
      frame True {
        # "Mean radius of the Earth in meters"
        n229 = formula code="lat_new = lat_new*Pi/180;\nlat_old = lat_old*Pi/180;\nlong_new = long_new*Pi/180;\nlong_old = long_old*Pi/180;\nd = asin(sqrt(sin((lat_old-lat_new)/2)**2+cos(lat_new)*cos(lat_old)*sin((long_old-long_new)/2)**2));\nd = 2*d*r/1000;"("Pi"=3.141592653589793, "r"=6372795.0, "long_old"=w483, "long_new"=w482, "lat_old"=w481, "lat_new"=w480) -> ("d"=w479:dbl)
      }
    }
    n230 = Multiply(x=1000.0, y=w470) -> (x*y=w454:dbl)
    n231 = case shown="假" "reset odometer" {
      tunnel: w464 -> [w475 _]
      tunnel: w463 -> [w474 _]
      tunnel: w457 -> [_ w476]
      tunnel: w458 -> [_ w477]
      tunnel: [w475 w477] -> w461
      tunnel: [w474 w476] -> w462
      frame False {
      }
      frame True {
      }
    }
    n232 = Less Or Equal?(x=w454, y=10000.0) -> (x <= y?=w455:bool)
    n233 = case shown="真" w455 {
      tunnel: w454 -> [_ w473]
      frame False {
      }
      frame True {
        n234 = global write "NMEA过程全局变量.vi" "BDOdometer"(w473) -> ()
        "偏移量/米" <- w473
      }
    }
    n235 = Bundle("纬度"=w462, "经度"=w461) -> (→"浮标定位点":cluster{"纬度":dbl, "经度":dbl})  [unwired: 1 in]
    n236 = local read "Stop"() -> (w469:bool)
  }
  n237 = while {
    tunnel: w1 -> [_]
    stop <- FALSE stop-if-true
    n238 = local read "定位状态"() -> (w488:bool)
    n239 = global read "NMEA断电保存全局变量.vi" "BD移位报警设定值"() -> (w495:dbl)
    n240 = global read "NMEA过程全局变量.vi" "BDOdometer"() -> (w496:dbl)
    n241 = Wait (ms)(milliseconds to wait=u32 1000 ("等待时间（毫秒）")) -> ()  [unwired: 1 out]
    n242 = call <vilib>:"Boolean Crossing PtByPt.vi"("direction"=enum16{"either", "false-true", "true-false"}."true-false", "input"=w488) -> ("crossing"=w487:bool)  [unwired: 1 in]
    n243 = Greater?(x=w496, y=w495) -> (0:w493:bool)
    n244 = call <vilib>:"Boolean Crossing PtByPt.vi"("direction"=enum16{"either", "false-true", "true-false"}."false-true", "input"=w493) -> ("crossing"=w492:bool)  [unwired: 1 in]
    n245 = case shown="真" w487 {
      selector: w487 -> [_ w499]
      tunnel: "北斗通信异常" ("设备") -> [_ w498]
      frame False {
      }
      frame True {
        # "触发告警"
        n246 = call "触发环动报警入队列.vi"("报警内容"=w498) -> ()  [unwired: 11 in]
        n247 = global read "断电保存全局变量.vi" "监测配置输出"() -> (w500:T17)
        n248 = Bundle By Name(cluster=w500, "北斗输出.定位告警"=w499, "北斗输出.告警内容"=w498) -> (w501:T17)
        n249 = global write "断电保存全局变量.vi" "监测配置输出"(w501) -> ()
      }
    }
    n250 = case shown="真" w492 {
      selector: w492 -> [_ w503]
      tunnel: "北斗移位报警" ("设备") -> [_ w502]
      frame False {
      }
      frame True {
        # "触发告警"
        n251 = call "触发环动报警入队列.vi"("报警内容"=w502) -> ()  [unwired: 11 in]
        n252 = global read "断电保存全局变量.vi" "监测配置输出"() -> (w504:T17)
        n253 = Bundle By Name(cluster=w504, "北斗输出.定位告警"=w503, "北斗输出.告警内容"=w502) -> (w505:T17)
        n254 = global write "断电保存全局变量.vi" "监测配置输出"(w505) -> ()
      }
    }
  }
  n255 = Release Queue(queue=w50, error in (no error)=w51) -> ()  [unwired: 1 in, 3 out]
  n256 = Release Queue(queue=w71, error in (no error)=w72) -> ()  [unwired: 1 in, 3 out]
  n257 = VISA Close(VISA resource name=w69, error in (no error)=w68) -> (error out=w73:errorcluster)
  n258 = call <vilib>:"Clear Errors.vi"("error in (no error)"=w73) -> ()  [unwired: 5 in, 2 out]
  n259 = while {
    stop <- FALSE stop-if-true
    n260 = global read "NMEA断电保存全局变量.vi" "BD波特率"() -> (→"波特率":u32)
    n261 = global read "NMEA断电保存全局变量.vi" "BDVISA资源名称"() -> (→"串口":refnum<visa-resource-name>)
    n262 = Wait (ms)(milliseconds to wait=u32 1000 ("等待时间（毫秒）")) -> ()  [unwired: 1 out]
  }
